vi "MDIO host.vi"() -> ()   [LabVIEW 2015]
uses:
  <vilib>/rvi/interface/nirviCloseFPGA/nirviCloseFPGA.xnode
  <vilib>/rvi/interface/nirviOpenFPGA/nirviOpenFPGA.xnode
  <vilib>/rvi/interface/nirviReadWriteControl/nirviReadWriteControl.xnode
  <vilib>/rvi/interface/Simulation/niFpgaSimulationCallBeginRW.vi
  <vilib>/rvi/errors/niLvFpgaAdjustHostInterfaceError.vi
  F:/FPGA ethernet/FPGA Bitfiles/FPGA_FPGATarget_MDIO_qvOKDtjQsAQ.lvbitx
  F:/FPGA ethernet/MDIO.vi
  <vilib>/FPGAPlugInAG/Dynamic/niLvFpga_Close_Dynamic.vi
panel:
  in  "OFF time, ms":u32
  in  "ON time, ms":u32
  in  "Enable":bool
  out "STATUS1_2":bool
  out "STATUS0_2":bool
  out "INIT/INT2":bool
  out "LOS2":bool
  in  "PWRDN2":bool
  in  "RESET2":bool
  out "STATUS1_1":bool
  out "STATUS0_1":bool
  out "INIT/INT1":bool
  out "LOS1":bool
  in  "PWRDN1":bool
  in  "RESET1":bool
  in  "Данные для записи":u16[](array[numeric])
  in  "Mode":u16(ring) items=["Packet generator", "Registers test"]
  out "Считанные данные":u16[](array[numeric])
  in  "PHY addr":u8
  in  "Write'n'read":bool
  in  "WaitUntilReadData":u32
  in  "AfterZDelay":u32
  # "1 - Режим сна"
  # "Registers test"
  # "Page 0, Register 9\nPage 0, Register 16\nPage 0, Register 26\nPage 0, Register 18\nPage 1, Register 16\nPage 1, Register 26\nPage 2, Register 16\nPage 3, Register 16\nPage 3, Register 17\nPage 3, Register 18\nPage 6, Register 16"
  # "Packet generator"
  # "При нажатой кнопке в цикле включается и отключается на заданное время (чтобы не завис wireshark)"
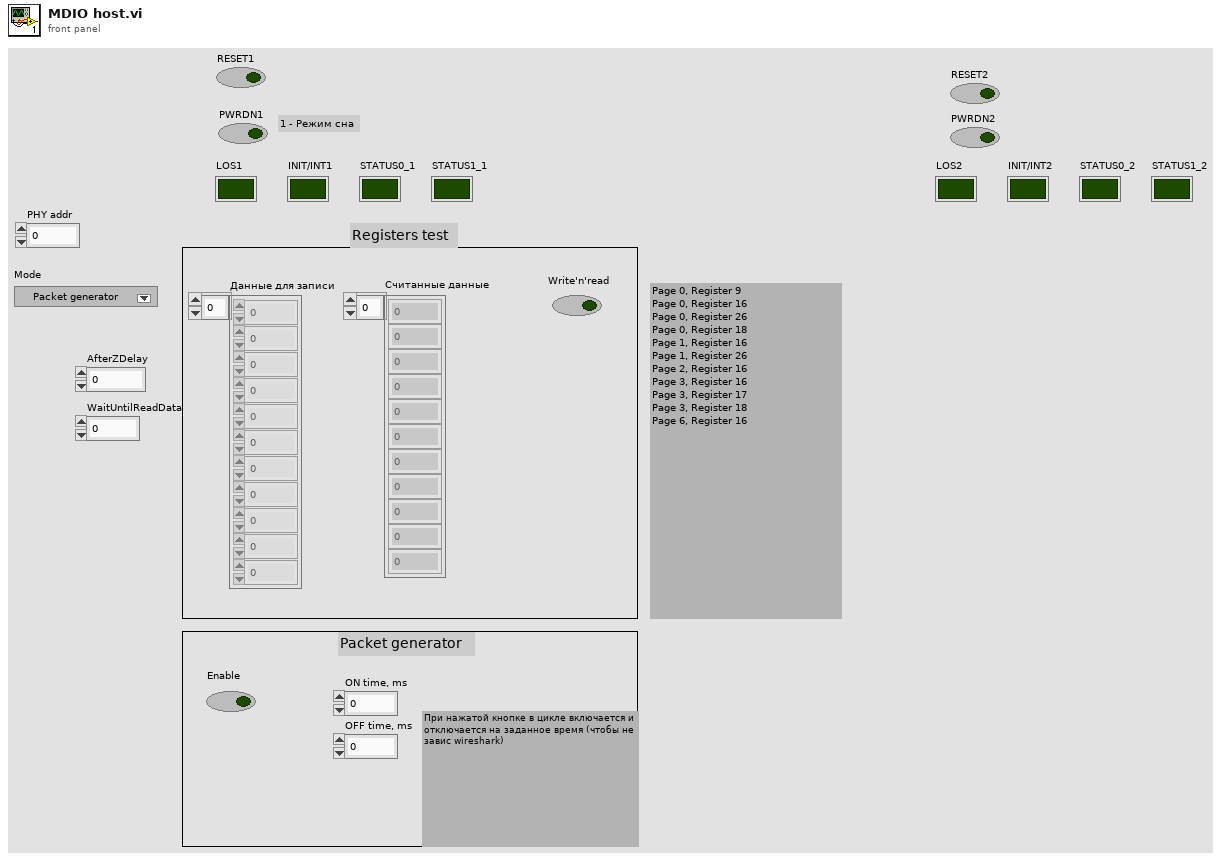
[diagram p1: front panel]
types:
  T1 = cluster{u16, u16, u16, u16, u16, u16, u16, u16, u16, u16, u16}
  T2 = cluster{u8, u8, u8, u8, u8, u8, u8, u8, u8, u8, u8}
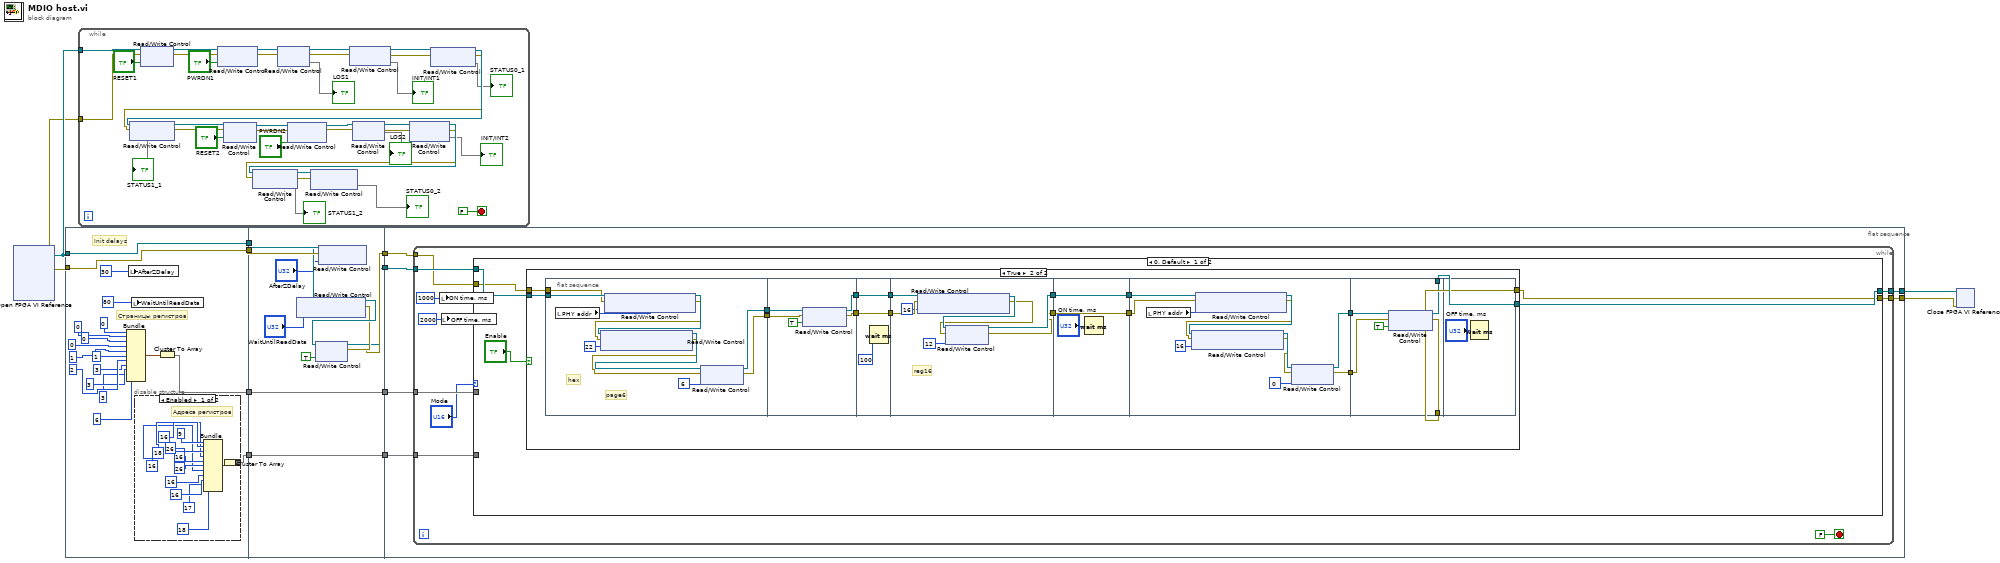
[diagram p0: block diagram]
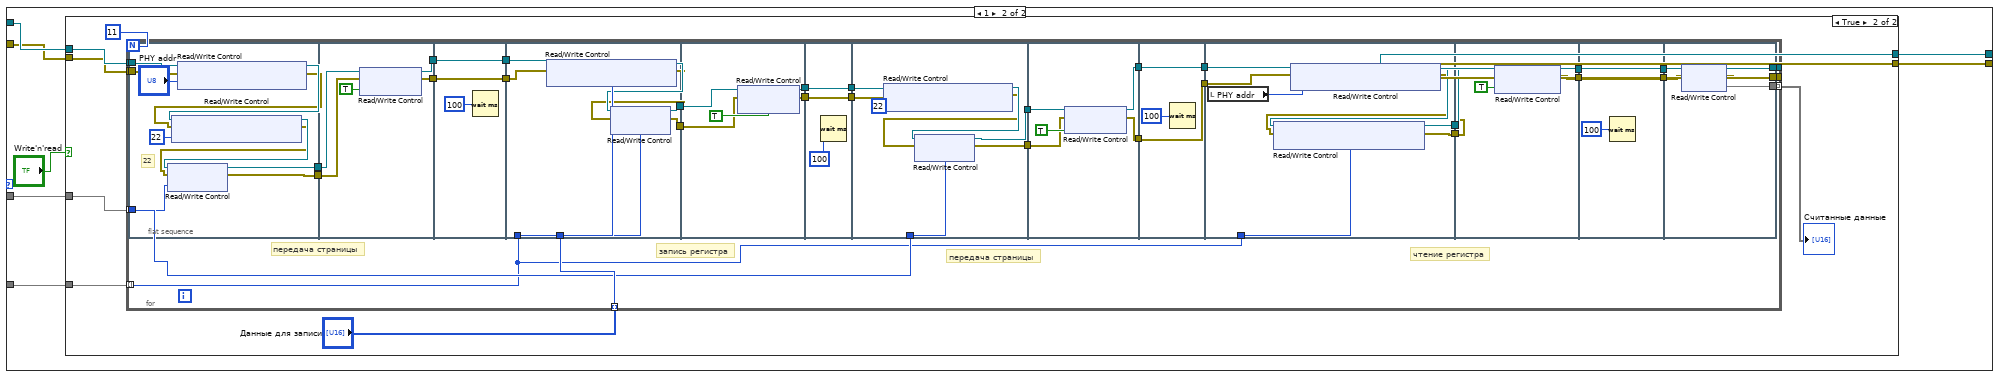
[diagram p4: hidden frame]
diagram:
  n1 = xnode "Open FPGA VI Reference"() -> ("FPGA VI Reference Out"=w3:refnum<k20>, "error out"=w2:errorcluster)  [unwired: 2 in]
  n2 = flat-sequence {
    tunnel: w3 -> [w30]
    tunnel: w2 -> [w29]
    tunnel: [w30] -> w12
    tunnel: [w29] -> w11
    tunnel: [w14] -> w8
    tunnel: [w13] -> w4
    tunnel: w12 -> [w56]
    tunnel: w11 -> [w55]
    tunnel: [w45] -> w10
    tunnel: [w50] -> w9
    tunnel: w8 -> [w50]
    tunnel: [w49] -> w5
    tunnel: w4 -> [w49]
    tunnel: [w44] -> w1
    tunnel: w10 -> [w61]
    tunnel: w9 -> [w60]
    tunnel: [w59] -> w7
    tunnel: [w58] -> w6
    tunnel: w5 -> [w57]
    tunnel: w1 -> [w62]
    frame #0 {
      # "Страницы регистров"
      # "Init delays"
      n3 = Bundle(u16 0, u16 0, u16 0, u16 0, u16 1, u16 1, u16 2, u16 3, u16 3, u16 3, u16 6) -> (w15:T1)  [unwired: 1 in]
      n4 = local write "AfterZDelay"(i16 30 ("DataPeriodDelay")) -> ()
      n5 = local write "WaitUntilReadData"(i16 80 ("DataPeriodDelay 2")) -> ()
      n6 = disable-structure shown="Enabled" {
        disable-tunnel: [w31 _] -> w13
        frame Enabled {
          # "Адреса регистров"
          n7 = Bundle(u8 9, u8 16, u8 26, u8 18, u8 16, u8 26, u8 16, u8 16, u8 16, u8 17, u8 18) -> (w32:T2)  [unwired: 1 in]
          n8 = Cluster To Array(cluster=w32) -> (array=w31:u8[])
        }
        frame Disabled {
        }
      }
      n9 = Cluster To Array(cluster=w15) -> (array=w14:u16[])
    }
    frame #1 {
      n10 = xnode "Read/Write Control"("FPGA VI Reference In"=w56, "error in"=w55, "AfterZDelay"="AfterZDelay") -> ("FPGA VI Reference Out"=w54:refnum<k20>, "error out"=w53:errorcluster)
      n11 = xnode "Read/Write Control"("FPGA VI Reference In"=w54, "error in"=w53, "WaitUntilReadData"="WaitUntilReadData") -> ("FPGA VI Reference Out"=w48:refnum<k20>, "error out"=w47:errorcluster)
      n12 = xnode "Read/Write Control"("FPGA VI Reference In"=w48, "error in"=w47, "Clock"=TRUE) -> ("FPGA VI Reference Out"=w44:refnum<k20>, "error out"=w45:errorcluster)
    }
    frame #2 {
      n13 = while {
        tunnel: w62 -> [w71]
        tunnel: w61 -> [w70]
        tunnel: w60 -> [w69]
        tunnel: [w68] -> w59
        tunnel: [w67] -> w58
        tunnel: w57 -> [w65]
        stop <- FALSE stop-if-true
        n14 = local write "ON time, ms"(u32 1000 ("ON time, ms")) -> ()
        n15 = local write "OFF time, ms"(u16 2000) -> ()
        n16 = case shown="0, Default" "Mode" {
          tunnel: w71 -> [w77 w149]
          tunnel: w70 -> [w76 w148]
          tunnel: w69 -> [_ w147]
          tunnel: [w74 w146] -> w68
          tunnel: [w73 w145] -> w67
          tunnel: w65 -> [_ w143]
          frame 0, Default {
            n17 = case shown="True" "Enable" {
              tunnel: w77 -> [w78 w93]
              tunnel: w76 -> [w79 w92]
              tunnel: [w79 w86] -> w73
              tunnel: [w78 w87] -> w74
              frame False {
              }
              frame True {
                n18 = flat-sequence {
                  tunnel: w93 -> [w106]
                  tunnel: w92 -> [w105]
                  tunnel: [w98] -> w95
                  tunnel: [w97] -> w94
                  tunnel: w95 -> [w110]
                  tunnel: w94 -> [w109]
                  tunnel: [w108] -> w83
                  tunnel: [w107] -> w81
                  tunnel: w83 -> [w114]
                  tunnel: [w114] -> w82
                  tunnel: w81 -> [w113]
                  tunnel: [w113] -> w80
                  tunnel: w82 -> [w121]
                  tunnel: w80 -> [w120]
                  tunnel: [w116] -> w85
                  tunnel: [w117] -> w84
                  tunnel: [w125] -> w91
                  tunnel: w85 -> [w124]
                  tunnel: [w124] -> w90
                  tunnel: w84 -> [w125]
                  tunnel: w91 -> [w134]
                  tunnel: w90 -> [w133]
                  tunnel: [w128] -> w89
                  tunnel: [w127] -> w88
                  tunnel: w89 -> [w140]
                  tunnel: w88 -> [w139]
                  tunnel: [w138] -> w87
                  tunnel: [w137] -> w86
                  frame #0 {
                    # "page6"
                    # "hex"
                    n19 = local read "PHY addr"() -> (w104:u8)
                    n20 = xnode "Read/Write Control"("FPGA VI Reference In"=w106, "error in"=w105, "Address (3 нуля первые)"=w104) -> ("FPGA VI Reference Out"=w103:refnum<k20>, "error out"=w102:errorcluster)
                    n21 = xnode "Read/Write Control"("FPGA VI Reference In"=w103, "error in"=w102, "RegAddr (3 нуля первые)"=u8 22) -> ("FPGA VI Reference Out"=w101:refnum<k20>, "error out"=w99:errorcluster)
                    n22 = xnode "Read/Write Control"("FPGA VI Reference In"=w101, "error in"=w99, "Data 16bit"=u16 6) -> ("FPGA VI Reference Out"=w98:refnum<k20>, "error out"=w97:errorcluster)
                  }
                  frame #1 {
                    n23 = xnode "Read/Write Control"("FPGA VI Reference In"=w110, "error in"=w109, "Transmit 1"=TRUE ("ReadData 1")) -> ("FPGA VI Reference Out"=w108:refnum<k20>, "error out"=w107:errorcluster)
                  }
                  frame #2 {
                    n24 = Wait (ms)(milliseconds to wait=u32 100) -> ()  [unwired: 1 out]
                  }
                  frame #3 {
                    # "reg16"
                    n25 = xnode "Read/Write Control"("FPGA VI Reference In"=w121, "error in"=w120, "RegAddr (3 нуля первые)"=u8 16) -> ("FPGA VI Reference Out"=w119:refnum<k20>, "error out"=w118:errorcluster)
                    n26 = xnode "Read/Write Control"("FPGA VI Reference In"=w119, "error in"=w118, "Data 16bit"=u16 12) -> ("FPGA VI Reference Out"=w117:refnum<k20>, "error out"=w116:errorcluster)
                  }
                  frame #4 {
                    n27 = Wait (ms)(milliseconds to wait="ON time, ms") -> ()  [unwired: 1 out]
                  }
                  frame #5 {
                    n28 = local read "PHY addr"() -> (w136:u8)
                    n29 = xnode "Read/Write Control"("FPGA VI Reference In"=w134, "error in"=w133, "Address (3 нуля первые)"=w136) -> ("FPGA VI Reference Out"=w132:refnum<k20>, "error out"=w131:errorcluster)
                    n30 = xnode "Read/Write Control"("FPGA VI Reference In"=w132, "error in"=w131, "RegAddr (3 нуля первые)"=u8 16) -> ("FPGA VI Reference Out"=w130:refnum<k20>, "error out"=w129:errorcluster)
                    n31 = xnode "Read/Write Control"("FPGA VI Reference In"=w130, "error in"=w129, "Data 16bit"=u16 0) -> ("FPGA VI Reference Out"=w128:refnum<k20>, "error out"=w127:errorcluster)
                  }
                  frame #6 {
                    n32 = xnode "Read/Write Control"("FPGA VI Reference In"=w140, "error in"=w139, "Transmit 1"=TRUE ("ReadData 1")) -> ("FPGA VI Reference Out"=w138:refnum<k20>, "error out"=w137:errorcluster)
                  }
                  frame #7 {
                    n33 = Wait (ms)(milliseconds to wait="OFF time, ms") -> ()  [unwired: 1 out]
                  }
                }
              }
            }
          }
          frame 1 {
            n34 = case shown="True" "Write'n'read" {
              tunnel: w149 -> [w151 w159]
              tunnel: w148 -> [w150 w158]
              tunnel: w147 -> [_ w157]
              tunnel: [w151 w155] -> w146
              tunnel: [w150 w154] -> w145
              tunnel: w143 -> [_ w153]
              frame False {
              }
              frame True {
                n35 = for {
                  N: 11 -> [_]
                  tunnel: w159 -> [w192]
                  tunnel: w158 -> [w191]
                  tunnel: w157 -> [w168] mode=indexing
                  tunnel: [w182] -> w156 mode=indexing
                  tunnel: [w184] -> w155
                  tunnel: [w183] -> w154
                  tunnel: w153 -> [w165] mode=indexing
                  tunnel: "Данные для записи" -> [w175] mode=indexing
                  # "чтение регистра"
                  # "передача страницы"
                  # "запись регистра"
                  # "передача страницы"
                  n36 = flat-sequence {
                    tunnel: w192 -> [w203]
                    tunnel: w191 -> [w202]
                    tunnel: [w195] -> w190
                    tunnel: [w194] -> w189
                    tunnel: w168 -> [w193]
                    tunnel: w190 -> [w207]
                    tunnel: w189 -> [w206]
                    tunnel: [w205] -> w188
                    tunnel: [w204] -> w187
                    tunnel: [w210] -> w177
                    tunnel: w188 -> [w210]
                    tunnel: w187 -> [w209]
                    tunnel: [w209] -> w176
                    tunnel: w177 -> [w219]
                    tunnel: w176 -> [w218]
                    tunnel: w165 -> [w217]
                    tunnel: w175 -> [w214]
                    tunnel: [w213] -> w174
                    tunnel: [w212] -> w173
                    tunnel: w174 -> [w223]
                    tunnel: w173 -> [w222]
                    tunnel: [w221] -> w171
                    tunnel: [w220] -> w169
                    tunnel: [w226] -> w172
                    tunnel: w171 -> [w226]
                    tunnel: [w225] -> w170
                    tunnel: w169 -> [w225]
                    tunnel: w172 -> [w235]
                    tunnel: w170 -> [w234]
                    tunnel: w168 -> [w230]
                    tunnel: [w229] -> w167
                    tunnel: [w228] -> w166
                    tunnel: w167 -> [w239]
                    tunnel: w166 -> [w238]
                    tunnel: [w237] -> w163
                    tunnel: [w236] -> w162
                    tunnel: [w242] -> w164
                    tunnel: w163 -> [w242]
                    tunnel: w162 -> [w241]
                    tunnel: [w241] -> w161
                    tunnel: [w248] -> w186
                    tunnel: [w247] -> w185
                    tunnel: w165 -> [w246]
                    tunnel: w164 -> [w245]
                    tunnel: w161 -> [w244]
                    tunnel: w186 -> [w256]
                    tunnel: w185 -> [w255]
                    tunnel: [w253] -> w181
                    tunnel: [w252] -> w179
                    tunnel: w181 -> [w259]
                    tunnel: [w259] -> w180
                    tunnel: w179 -> [w258]
                    tunnel: [w258] -> w178
                    tunnel: w180 -> [w264]
                    tunnel: w178 -> [w263]
                    tunnel: [w262] -> w182
                    tunnel: [w261] -> w184
                    tunnel: [w260] -> w183
                    frame #0 {
                      # "22"
                      n37 = xnode "Read/Write Control"("FPGA VI Reference In"=w203, "error in"=w202, "Address (3 нуля первые)"="PHY addr") -> ("FPGA VI Reference Out"=w200:refnum<k20>, "error out"=w199:errorcluster)
                      n38 = xnode "Read/Write Control"("FPGA VI Reference In"=w200, "error in"=w199, "RegAddr (3 нуля первые)"=u8 22) -> ("FPGA VI Reference Out"=w197:refnum<k20>, "error out"=w196:errorcluster)
                      n39 = xnode "Read/Write Control"("FPGA VI Reference In"=w197, "error in"=w196, "Data 16bit"=w193) -> ("FPGA VI Reference Out"=w195:refnum<k20>, "error out"=w194:errorcluster)
                    }
                    frame #1 {
                      n40 = xnode "Read/Write Control"("FPGA VI Reference In"=w207, "error in"=w206, "Transmit 1"=TRUE ("ReadData 1")) -> ("FPGA VI Reference Out"=w205:refnum<k20>, "error out"=w204:errorcluster)
                    }
                    frame #2 {
                      n41 = Wait (ms)(milliseconds to wait=u32 100) -> ()  [unwired: 1 out]
                    }
                    frame #3 {
                      n42 = xnode "Read/Write Control"("FPGA VI Reference In"=w219, "error in"=w218, "RegAddr (3 нуля первые)"=w217) -> ("FPGA VI Reference Out"=w216:refnum<k20>, "error out"=w215:errorcluster)
                      n43 = xnode "Read/Write Control"("FPGA VI Reference In"=w216, "error in"=w215, "Data 16bit"=w214) -> ("FPGA VI Reference Out"=w213:refnum<k20>, "error out"=w212:errorcluster)
                    }
                    frame #4 {
                      n44 = xnode "Read/Write Control"("FPGA VI Reference In"=w223, "error in"=w222, "Transmit 1"=TRUE ("ReadData 1")) -> ("FPGA VI Reference Out"=w221:refnum<k20>, "error out"=w220:errorcluster)
                    }
                    frame #5 {
                      n45 = Wait (ms)(milliseconds to wait=u32 100) -> ()  [unwired: 1 out]
                    }
                    frame #6 {
                      n46 = xnode "Read/Write Control"("FPGA VI Reference In"=w235, "error in"=w234, "RegAddr (3 нуля первые)"=u8 22) -> ("FPGA VI Reference Out"=w232:refnum<k20>, "error out"=w231:errorcluster)
                      n47 = xnode "Read/Write Control"("FPGA VI Reference In"=w232, "error in"=w231, "Data 16bit"=w230) -> ("FPGA VI Reference Out"=w229:refnum<k20>, "error out"=w228:errorcluster)
                    }
                    frame #7 {
                      n48 = xnode "Read/Write Control"("FPGA VI Reference In"=w239, "error in"=w238, "Transmit 1"=TRUE ("ReadData 1")) -> ("FPGA VI Reference Out"=w237:refnum<k20>, "error out"=w236:errorcluster)
                    }
                    frame #8 {
                      n49 = Wait (ms)(milliseconds to wait=u32 100) -> ()  [unwired: 1 out]
                    }
                    frame #9 {
                      n50 = local read "PHY addr"() -> (w251:u8)
                      n51 = xnode "Read/Write Control"("FPGA VI Reference In"=w245, "error in"=w244, "ReadAddress (3 нуля первые)"=w251) -> ("FPGA VI Reference Out"=w250:refnum<k20>, "error out"=w249:errorcluster)
                      n52 = xnode "Read/Write Control"("FPGA VI Reference In"=w250, "error in"=w249, "ReadRegAddr (3 нуля первые)"=w246) -> ("FPGA VI Reference Out"=w248:refnum<k20>, "error out"=w247:errorcluster)
                    }
                    frame #10 {
                      n53 = xnode "Read/Write Control"("FPGA VI Reference In"=w256, "error in"=w255, "ReadData 1"=TRUE) -> ("FPGA VI Reference Out"=w253:refnum<k20>, "error out"=w252:errorcluster)
                    }
                    frame #11 {
                      n54 = Wait (ms)(milliseconds to wait=u32 100) -> ()  [unwired: 1 out]
                    }
                    frame #12 {
                      n55 = xnode "Read/Write Control"("FPGA VI Reference In"=w264, "error in"=w263) -> ("FPGA VI Reference Out"=w261:refnum<k20>, "error out"=w260:errorcluster, "Data"=w262)
                    }
                  }
                }
                "Считанные данные" <- w156
              }
            }
          }
        }
      }
    }
  }
  n56 = while {
    tunnel: w3 -> [w300]
    tunnel: w2 -> [w299]
    stop <- FALSE stop-if-true
    n57 = xnode "Read/Write Control"("FPGA VI Reference In"=w300, "error in"=w299, "RESET1"="RESET1") -> ("FPGA VI Reference Out"=w298:refnum<k20>, "error out"=w297:errorcluster)
    n58 = xnode "Read/Write Control"("FPGA VI Reference In"=w298, "error in"=w297, "PWRDN1"="PWRDN1") -> ("FPGA VI Reference Out"=w294:refnum<k20>, "error out"=w293:errorcluster)
    n59 = xnode "Read/Write Control"("FPGA VI Reference In"=w294, "error in"=w293) -> ("FPGA VI Reference Out"=w292:refnum<k20>, "error out"=w291:errorcluster, "LOS1"=→"LOS1")
    n60 = xnode "Read/Write Control"("FPGA VI Reference In"=w292, "error in"=w291) -> ("FPGA VI Reference Out"=w290:refnum<k20>, "error out"=w289:errorcluster, "INIT/INT1"=→"INIT/INT1")
    n61 = xnode "Read/Write Control"("FPGA VI Reference In"=w290, "error in"=w289) -> ("FPGA VI Reference Out"=w287:refnum<k20>, "error out"=w286:errorcluster, "STATUS0_1"=→"STATUS0_1")
    n62 = xnode "Read/Write Control"("FPGA VI Reference In"=w287, "error in"=w286) -> ("FPGA VI Reference Out"=w283:refnum<k20>, "error out"=w282:errorcluster, "STATUS1_1"=→"STATUS1_1")
    n63 = xnode "Read/Write Control"("FPGA VI Reference In"=w283, "error in"=w282, "RESET2"="RESET2") -> ("FPGA VI Reference Out"=w280:refnum<k20>, "error out"=w279:errorcluster)
    n64 = xnode "Read/Write Control"("FPGA VI Reference In"=w280, "error in"=w279, "PWRDN2"="PWRDN2") -> ("FPGA VI Reference Out"=w277:refnum<k20>, "error out"=w276:errorcluster)
    n65 = xnode "Read/Write Control"("FPGA VI Reference In"=w277, "error in"=w276) -> ("FPGA VI Reference Out"=w275:refnum<k20>, "error out"=w274:errorcluster, "LOS2"=→"LOS2")
    n66 = xnode "Read/Write Control"("FPGA VI Reference In"=w275, "error in"=w274) -> ("FPGA VI Reference Out"=w273:refnum<k20>, "error out"=w270:errorcluster, "INIT/INT2"=→"INIT/INT2")
    n67 = xnode "Read/Write Control"("FPGA VI Reference In"=w273, "error in"=w270) -> ("FPGA VI Reference Out"=w272:refnum<k20>, "error out"=w271:errorcluster, "STATUS1_2"=→"STATUS1_2")
    n68 = xnode "Read/Write Control"("FPGA VI Reference In"=w272, "error in"=w271) -> ("STATUS0_2"=→"STATUS0_2")  [unwired: 2 out]
  }
  n69 = xnode "Close FPGA VI Reference"("FPGA VI Reference In"=w7, "error in"=w6) -> ()  [unwired: 1 out]
